vi "Delete.vi"(8 "error in (no error)":errorcluster, 10 "Path":string, 11 "SCP File Transfer in":refnum<class "SCP File Transfer.lvclass">) -> (0 "error out":errorcluster, 3 "SCP File Transfer out":refnum<class "SCP File Transfer.lvclass">)   [LabVIEW 2013, in "PL Framework Configuration Tool.lvlib" / "SCP File Transfer.lvclass"]
doc: "Deletes a file or empty directory located at \"Path\".\n\nIf you wish to delete a directory, it is recommended you use \"Delete directory.vi\", as it can handle non-empty directories and can also delete only the directory contents and not the directory itself."
uses:
  SCP File Transfer.lvclass
  <vilib>/NI/RT Management/classes/File Transfer Behavior/File Transfer Behavior.lvclass
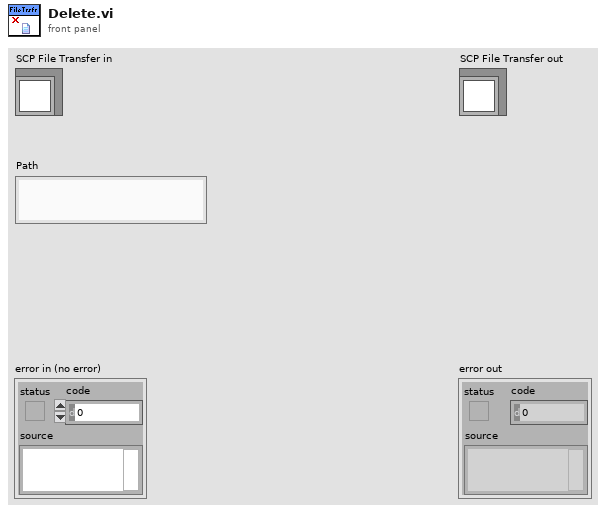
[diagram p1: front panel]
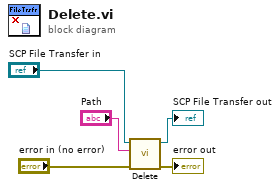
[diagram p0: block diagram]
diagram:
  n1 = call-parent "Delete.vi"("error in (no error)"="error in (no error)", "Path"="Path", "File Transfer Behavior in"="SCP File Transfer in") -> ("error out"=→"error out":errorcluster, "File Transfer Behavior out"=→"SCP File Transfer out":refnum<class "SCP File Transfer.lvclass">)  [unwired: 7 in]
